vi "PH_gentec_P-Link.Action open connection.vi"(0 "i ref in":refnum<vi>, 2 "VISA resource in":refnum<visa-resource-name>, 5 "error in":errorcluster) -> (14 "i ref out":refnum<vi>, 19 "error out":errorcluster)   [LabVIEW 2014, in "PH_gentec_P-Link.lvlib"]
doc: "This VI opens the VISA connection."
uses:
  PH_gentec_P-Link.lvlib
  PH_Basics/PH_Powermeter_BaseClass/PH_Powermeter_BaseClass.State.ctl
  PH_Basics/PH_Powermeter_BaseClass/PH_Powermeter_BaseClass.Connection.ctl
  PH_Basics/PH_Powermeter_BaseClass/PH_Powermeter_BaseClass.lvlib
  instr.lib/Gentec-P-Link/gentec-P-Link - Driver.lvlib
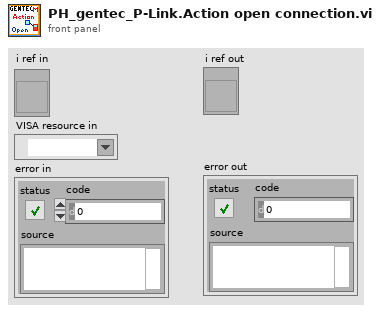
[diagram p1: front panel]
types:
  T1 = typedef "PH_Powermeter_BaseClass.lvlib/PH_Powermeter_BaseClass.Connection.ctl" = cluster{"failed checks":i8, "Timeout":bool, "Data read":string, "Failure":bool, "Error":bool, "State":T2}
  T2 = typedef "PH_Powermeter_BaseClass.lvlib/PH_Powermeter_BaseClass.State.ctl" = enum32{"off", "operating", "opened", "checked", "connected", "Sets to change", "running"}
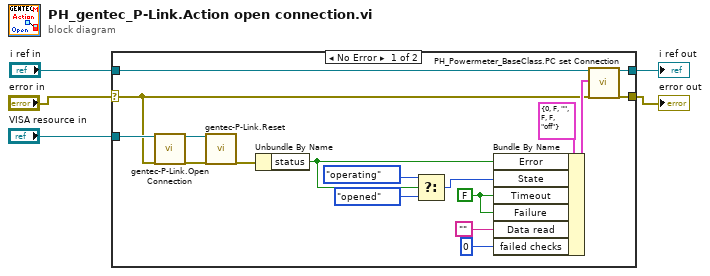
[diagram p0: block diagram]
diagram:
  n1 = case shown="No Error" "error in" {
    selector: "error in" -> [w9 w24]
    tunnel: [w11 w24] -> w5
    tunnel: "VISA resource in" -> [w10 _]
    tunnel: "i ref in" -> [w15 w23]
    tunnel: [w12 w23] -> w1
    frame No Error {
      w21 = FALSE ("Connection.Timeout")
      n2 = call "gentec-P-Link.Open Connection.vi"("VISA resource name"=w10, "error in (no error)"=w9) -> ("VISA resource name"=w6:refnum<visa-resource-name>, "error out"=w8:errorcluster)  [unwired: 16 in]
      n3 = call "gentec-P-Link.Reset.vi"("VISA resource name"=w6, "error in (no error)"=w8) -> ("error out"=w7:errorcluster)  [unwired: 16 in, 1 out]
      n4 = Unbundle By Name(w7) -> ("status"=w20:bool)
      n5 = Select(t=PH_Powermeter_BaseClass.State."operating" ("State"), s=w20, f=PH_Powermeter_BaseClass.State."opened") -> (s? t:f=w17:T2)
      n6 = Bundle By Name(cluster=T1 {"failed checks"=0, "Timeout"=FALSE, "Data read"="", "Failure"=FALSE, "Error"=FALSE, "State"=enum."off"} ("Connection in"), "Error"=w20, "State"=w17, "Timeout"=w21, "Failure"=w21, "Data read"="", "failed checks"=i8 0) -> (w13:T1)
      n7 = call "PH_Powermeter_BaseClass.PC set Connection.vi"("VI in"=w15, "Connection"=w13, "error in (no error)"=w9) -> ("VI out"=w12:refnum<vi>, "error out"=w11:errorcluster)  [unwired: 15 in]
    }
    frame Error {
    }
  }
  "error out" <- w5
  "i ref out" <- w1
